vi "SV Multitone SINAD and THD+N.vi"   [LabVIEW 2017, in "SoundVib_Multitone.lvlib"]
doc: "Performs a signal in noise and distortion (SINAD) analysis and analyzes total harmonic distortion plus noise (THD + N), including measuring the fundamental tones, and returns the and SINAD and THD + N in the desired units. Wire data to the <B>scaled signal [EU]</B> input to determine the polymorphic instance to use or manually select the instance.\n\nThe following formula calculates SINAD:\n\nSINAD = sqrt(F2 + N2 + H2) / sqrt(H2 + N2)\n\nwhere F is the fundamental tone RMS level, N is the noise RMS level, and H is the harmonic RMS level."
uses:
  <vilib>/addons/Sound and Vibration/svt_Multitone Distortion/SoundVib_Multitone.lvlib
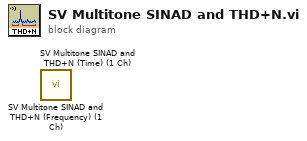
[diagram p0: block diagram]
diagram:
  n1 = call <vilib>:"SV Multitone SINAD and THD+N (Frequency) (1 Ch).vi"() -> ()  [unwired: 14 in, 6 out]
  n2 = call <vilib>:"SV Multitone SINAD and THD+N (Time) (1 Ch).vi"() -> ()  [unwired: 14 in, 6 out]
